vi "Status-Request-ServerInstance-Name.vi"(8 "error in (no error)":errorcluster, 9 "Response Timeout(5000ms)":i32=5000, 11 "connection ID":refnum<k5>) -> (0 "error IO":errorcluster, 2 "Server Instance Name":string, 3 "connection ID(dup)":refnum<k5>)   [LabVIEW 2020, in "CSM-TCP-Router.lvlib" / "TcpRouter-Client.lvclass"]
uses:
  TcpRouter-Client.lvclass
  _support/tcp-msg type.ctl
  f6a5f277-00bd-489a-a8fe-1f8d73284ee1.vi
  <userlib>/_NEVSTOP/Communicable State Machine(CSM)/AdvanceAPI/CSM - Revert Arguments-Safe String.vi
  <userlib>/_NEVSTOP/Communicable State Machine(CSM)/_Shared/Trim Single-line Text.vi
  <userlib>/_NEVSTOP/Communicable State Machine(CSM)/AdvanceAPI/CSM - Keywords.vi
  CSM-TCP-Router.lvlib
  <userlib>/_NEVSTOP/Communicable State Machine(CSM)/Communicable State Machine.lvlib
panel:
  # "Connector Pane"
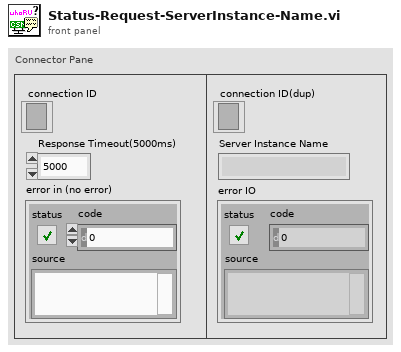
[diagram p1: front panel]
types:
  T1 = typedef "CSM-TCP-Router.lvlib/tcp-msg type.ctl" = enum8{"info", "error", "cmd", "cmd-resp", "resp", "async-resp", "status", "interrupt"}
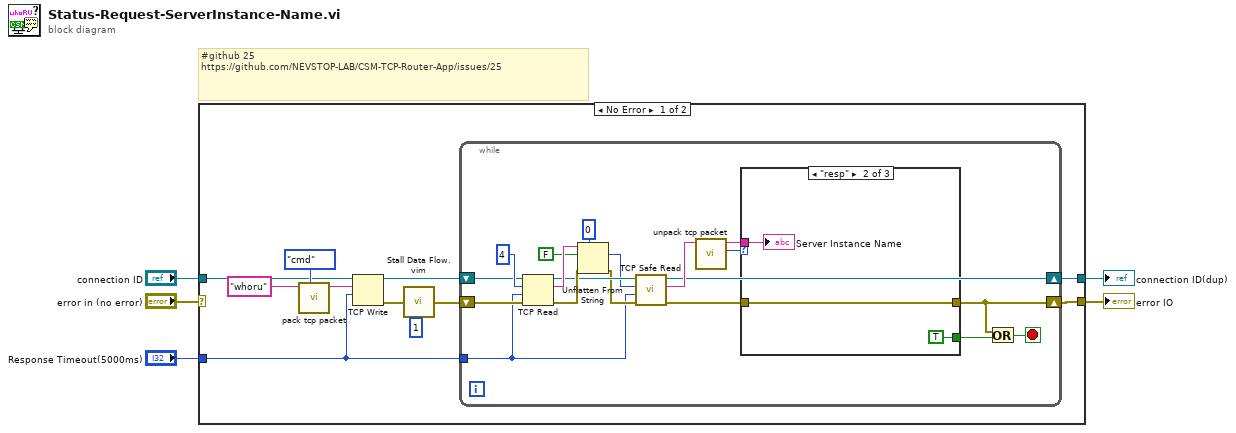
[diagram p0: block diagram]
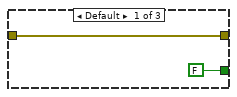
[diagram p2: hidden frame]
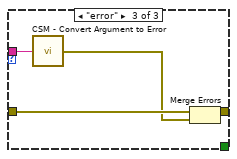
[diagram p3: hidden frame]
diagram:
  # "#github 25\nhttps://github.com/NEVSTOP-LAB/CSM-TCP-Router-App/issues/25"
  n1 = case shown="No Error" "error in (no error)" {
    selector: "error in (no error)" -> [_ w46]
    tunnel: "Response Timeout(5000ms)" -> [w10 _]
    tunnel: [w9 w46] -> w4
    tunnel: "connection ID" -> [w8 w45]
    tunnel: [w7 w45] -> w1
    frame No Error {
      n2 = call "pack tcp packet.vi"("tcp-message-type"=tcp-msg_type."cmd", "String"="whoru") -> ("TCP Pack"=w16:string)  [unwired: 9 in]
      n3 = TCP Write(connection ID=w8, data in=w16, 9:w10) -> (connection ID out=w12:refnum<k5>, error out=w14:errorcluster)  [unwired: 1 in, 1 out]
      n4 = call "Stall Data Flow.vim"("value in"=w14, "milliseconds to wait"=u32 1) -> ("value out"=w11:errorcluster)  [unwired: 1 out]
      n5 = while {
        tunnel: w10 -> [w21]
        shift-right: [w20] -> w7
        shift-left: w12 -> [w23]
        shift-right: [w18] -> w9
        shift-left: w11 -> [w22]
        stop <- w19 stop-if-true
        n6 = TCP Read(connection ID=w23, bytes to read=4, error in (no error)=w22, 9:w21) -> (connection ID out=w33:refnum<k5>, data out=w34:string, error out=w35:errorcluster)  [unwired: 1 in]
        n7 = Unflatten From String(type=0, binary string=w34, data includes array or string size? (T)=FALSE, error in (no error)=w35) -> (value=w31:i32, error out=w30:errorcluster)  [unwired: 2 out]
        n8 = call "TCP Safe Read.vi"("error in (no error)"=w30, "timeout ms (25000)"=w21, "bytes to read"=w31, "TCP Network Connection in"=w33) -> ("error out"=w25:errorcluster, "String"=w32:string, "TCP Network Connection out"=w20:refnum<k5>)  [unwired: 5 in]
        n9 = call "unpack tcp packet.vi"("TCP Pack"=w32) -> ("tcp-message-type"=w26:T1, "String"=w24:string)  [unwired: 9 in]
        n10 = case shown="\"resp\"" w26 {
          tunnel: w25 -> [w37 w39 w44]
          tunnel: [w37 w39 w42] -> w18
          tunnel: w24 -> [_ w40 w43]
          tunnel: [FALSE TRUE _] -> w17
          frame Default {
          }
          frame "resp" {
            "Server Instance Name" <- w40
          }
          frame "error" {
            n11 = call <userlib>:"CSM - Convert Argument to Error.vi"("Argument"=w43) -> ("Error"=w41:errorcluster)  [unwired: 4 in]
            n12 = Merge Errors(w44, w41) -> (w42:errorcluster)
          }
        }
        n13 = Or(x=w18, y=w17) -> (x .or. y?=w19:bool)
      }
    }
    frame Error {
    }
  }
  "error IO" <- w4
  "connection ID(dup)" <- w1
